vi "Synch with Server.vi"(10 "Sensor File Name":string, 11 "App Config":T1={"Support Dir (Local)"=path "C:/Users/gtetil/Documents/Projects/TI-cDAQ/Source/Support", "Support Dir (Remote)"=path "S:/GLOBALTEST/Software/TI cDAQ/Support", "Config Sub Dir"="Configurations", "Last Config (Std)"="", "Last Config (Def)"="", "Last Config (8TC)"=""}) -> (0 "Error OUT":errorcluster)   [LabVIEW 2023]
uses:
  Type Defs and Controls/App Config.ctl
  Type Defs and Controls/Sensor.ctl
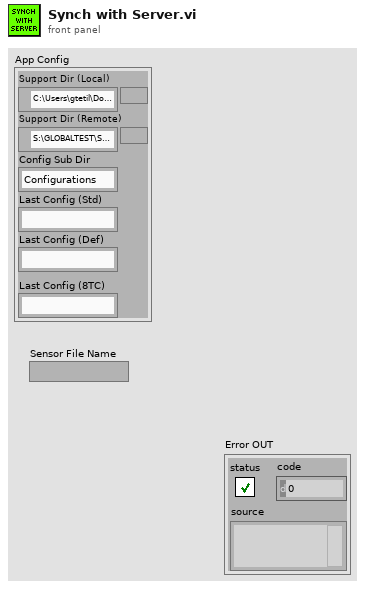
[diagram p1: front panel]
types:
  T1 = typedef "App Config.ctl" = cluster{"Support Dir (Local)":path, "Support Dir (Remote)":path, "Config Sub Dir":string, "Last Config (Std)":string, "Last Config (Def)":string, "Last Config (8TC)":string}
  T2 = typedef "Sensor.ctl" = cluster{"Sensor Name":string, "Sensor Info":cluster{"Manufacturer":string, "Model":string, "Serial Number":string}, "Last Cal Info":cluster{"Last Calibration Date":dbl, "Calibrator":string, "Cal Duration":i32}, "Voltage Range":cluster{"High Limit":dbl, "Low Limit":dbl}, "EGU Range":cluster{"High Limit":dbl, "Low Limit":dbl}, "Units":string, "Calibration Type":enum16{"Calibrate Analog", "Compare Analog Calibration"}, "EGU List":dbl[], "Voltage List":dbl[], "Coefficients":dbl[], "Order":i32, "Algorithm":enum32{"SVD", "Givens", "Givens2", "Householder", "LU Decomposition", "Cholesky"}, "Max Error % of Full Scale":dbl, "Max Mean Squared Error":dbl, "Use Error %":bool, "Use MSE":bool, "Allow Manual Entry":bool, "Max Stability Error":dbl, "Max Error % of Reading":dbl, "Use Error % of Reading":bool}
  T3 = enum16{"Left Button", "Center Button", "Right Button", "Window Close"}
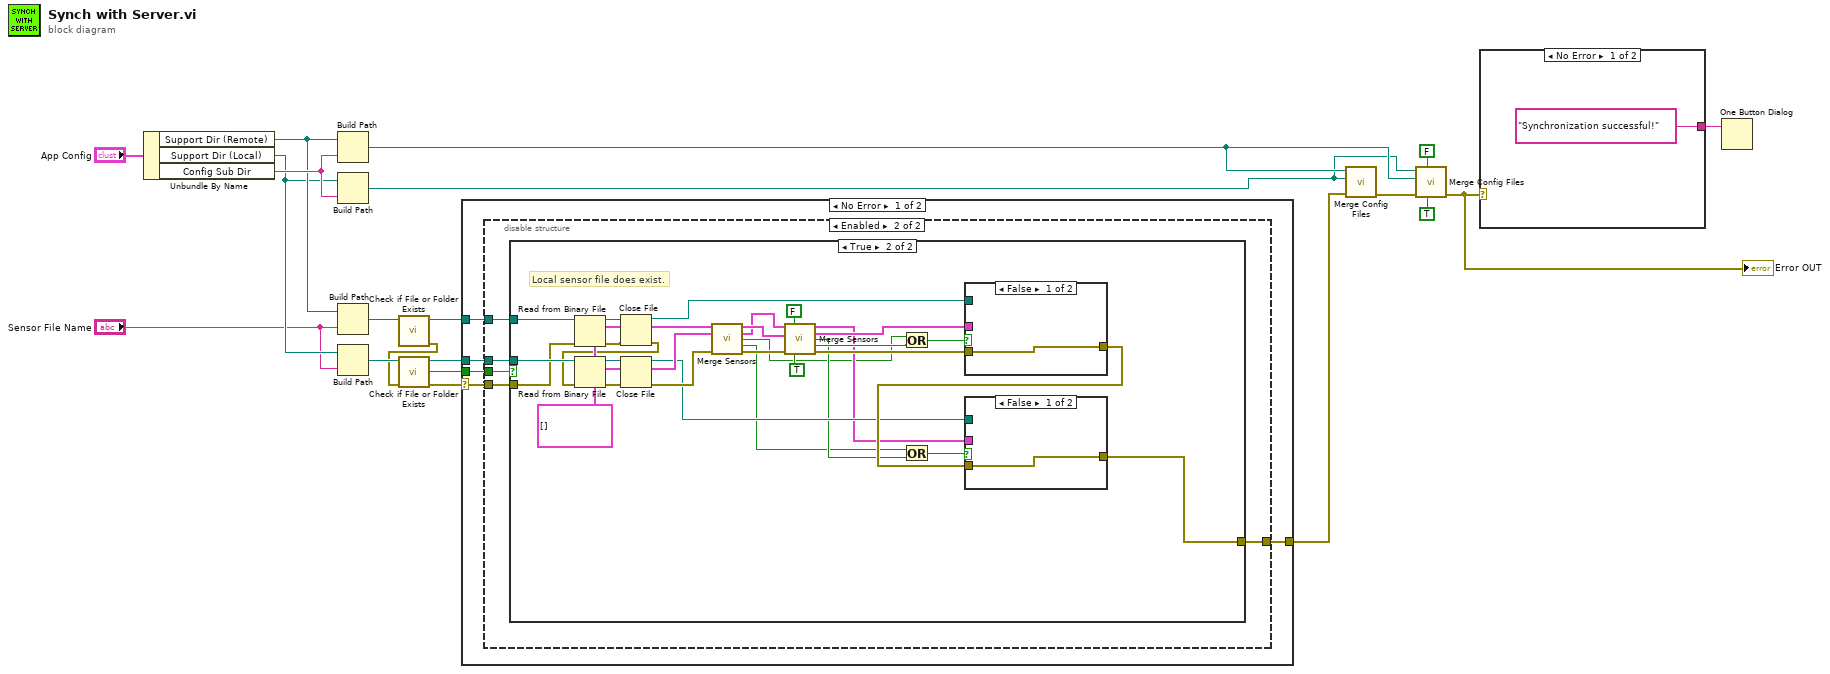
[diagram p0: block diagram]
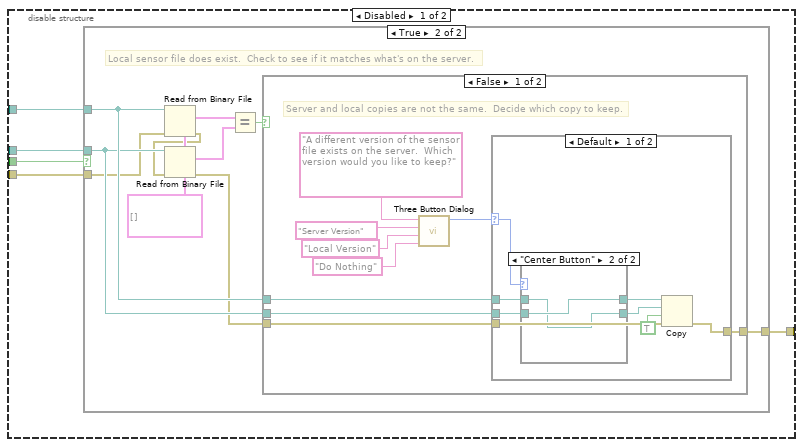
[diagram p2: hidden frame]
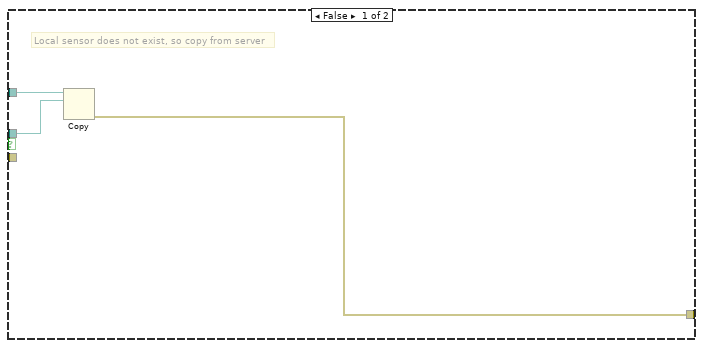
[diagram p3: hidden frame]
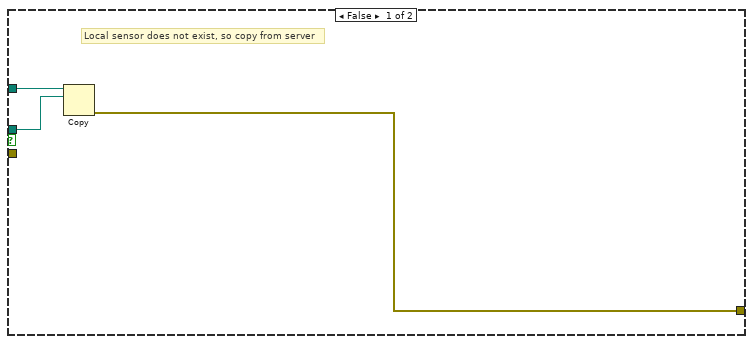
[diagram p7: hidden frame]
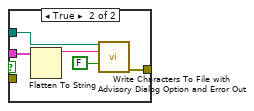
[diagram p8: hidden frame]
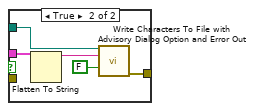
[diagram p9: hidden frame]
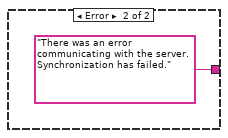
[diagram p11: hidden frame]
diagram:
  n1 = Unbundle By Name("App Config") -> ("Support Dir (Remote)"=w18:path, "Support Dir (Local)"=w17:path, "Config Sub Dir"=w19:string)
  n2 = Build Path(base path=w18, name or relative path=w19) -> (appended path=w15:path)
  n3 = Build Path(base path=w17, name or relative path=w19) -> (appended path=w14:path)
  n4 = Build Path(base path=w18, name or relative path="Sensor File Name") -> (appended path=w4:path)
  n5 = Build Path(base path=w17, name or relative path="Sensor File Name") -> (appended path=w11:path)
  n6 = call <vilib>:"Check if File or Folder Exists.vi"("path"=w4) -> ("error out"=w2:errorcluster, "dup path"=w3:path)  [unwired: 8 in, 1 out]
  n7 = call <vilib>:"Check if File or Folder Exists.vi"("error in (no error)"=w2, "path"=w11) -> ("error out"=w1:errorcluster, "file or folder exists?"=w10:bool, "dup path"=w9:path)  [unwired: 7 in]
  n8 = case shown="No Error" w1 {
    selector: w1 -> [w21 w117]
    tunnel: w10 -> [w25 _]
    tunnel: w9 -> [w24 _]
    tunnel: [w23 w117] -> w6
    tunnel: w3 -> [w22 _]
    frame No Error {
      n9 = disable-structure shown="Enabled" {
        disable-tunnel: w25 -> [w30 w71]
        disable-tunnel: w24 -> [w29 w70]
        disable-tunnel: [w28 w69] -> w23
        disable-tunnel: w22 -> [w27 w68]
        disable-tunnel: w21 -> [w26 w67]
        frame Disabled {
          n10 = case shown="True" w30 {
            tunnel: w27 -> [w33 w39]
            tunnel: w29 -> [w32 w38]
            tunnel: [w31 w37] -> w28
            tunnel: w26 -> [_ w36]
            frame False {
              # "Local sensor does not exist, so copy from server"
              n11 = Copy(10:w32, 11:w33) -> (0:w31:errorcluster)  [unwired: 3 in, 2 out]
            }
            frame True {
              w43 = T2[] [] ("Sensors")
              # "Local sensor file does exist.  Check to see if it matches what's on the server."
              n12 = Read from Binary File(5:w43, 8:w36, 11:w39) -> (0:w35:errorcluster, 2:w42:T2[])  [unwired: 3 in, 2 out]
              n13 = Read from Binary File(5:w43, 8:w35, 11:w38) -> (0:w34:errorcluster, 2:w41:T2[])  [unwired: 3 in, 2 out]
              n14 = Equal?(x=w42, y=w41) -> (x = y?=w40:bool)
              n15 = case shown="False" w40 {
                tunnel: w39 -> [w47 _]
                tunnel: w38 -> [w46 _]
                tunnel: [w45 w66] -> w37
                tunnel: w34 -> [w44 w66]
                frame False {
                  # "Server and local copies are not the same.  Decide which copy to keep."
                  n16 = call <vilib>:"Three Button Dialog.vi"("Right Button Text (\"Cancel\")"="Do Nothing" ("T button name (\"OK\")"), "Center Button Text (\"No\")"="Local Version" ("T button name (\"OK\")"), "Left Button Text (\"Yes\")"="Server Version" ("T button name (\"OK\")"), "message"="A different version of the sensor file exists on the server.  Which version would you like to keep?") -> ("Which Button?"=w48:T3)  [unwired: 7 in]
                  n17 = case shown="Default" w48 {
                    selector: w48 -> [w58 _]
                    tunnel: w47 -> [w57 _]
                    tunnel: [w60 w65] -> w45
                    tunnel: w46 -> [w55 _]
                    tunnel: w44 -> [w53 w65]
                    frame Default {
                      n18 = case shown="\"Center Button\"" w58 {
                        tunnel: [w62 w64] -> w56
                        tunnel: w57 -> [w62 w63]
                        tunnel: [w61 w63] -> w54
                        tunnel: w55 -> [w61 w64]
                        frame "Left Button", Default {
                        }
                        frame "Center Button" {
                        }
                      }
                      n19 = Copy(8:w53, 9:TRUE ("overwrite (F)"), 10:w54, 11:w56) -> (0:w60:errorcluster)  [unwired: 1 in, 2 out]
                    }
                    frame "Right Button" {
                    }
                  }
                }
                frame True {
                  # "Server and local copies are the same, so do nothing."
                }
              }
            }
          }
        }
        frame Enabled {
          n20 = case shown="True" w71 {
            tunnel: w68 -> [w74 w94]
            tunnel: w70 -> [w73 w103]
            tunnel: [w72 w91] -> w69
            tunnel: w67 -> [_ w102]
            frame False {
              # "Local sensor does not exist, so copy from server"
              n21 = Copy(10:w73, 11:w74) -> (0:w72:errorcluster)  [unwired: 3 in, 2 out]
            }
            frame True {
              w104 = T2[] [] ("Sensors")
              # "Local sensor file does exist."
              n22 = Read from Binary File(5:w104, 8:w102, 11:w94) -> (0:w89:errorcluster, 2:w100:T2[], 3:w90:refnum<file>)  [unwired: 3 in, 1 out]
              n23 = Close File(refnum=w90, error in=w89) -> (path=w84:path, error out=w88:errorcluster)
              n24 = Read from Binary File(5:w104, 8:w88, 11:w103) -> (0:w86:errorcluster, 2:w99:T2[], 3:w87:refnum<file>)  [unwired: 3 in, 1 out]
              n25 = Close File(refnum=w87, error in=w86) -> (path=w83:path, error out=w85:errorcluster)
              n26 = call "Merge Sensors.vi"("Source Sensors IN"=w100, "Dest Sensors IN"=w99, "Error IN"=w85) -> ("Source Sensors OUT"=w96:T2[], "Dest Sensors OUT"=w95:T2[], "Source Changed"=w76:bool, "Dest Changed"=w75:bool, "Error OUT"=w101:errorcluster)  [unwired: 8 in]
              n27 = call "Merge Sensors.vi"("Source Sensors IN"=w95, "Server is Source (T)"=FALSE, "Dest Sensors IN"=w96, "Error IN"=w101, "Version Prompt (F)"=TRUE) -> ("Source Sensors OUT"=w77:T2[], "Dest Sensors OUT"=w78:T2[], "Source Changed"=w79:bool, "Dest Changed"=w80:bool, "Error OUT"=w93:errorcluster)  [unwired: 6 in]
              n28 = Or(x=w76, y=w80) -> (x .or. y?=w82:bool)
              n29 = Or(x=w75, y=w79) -> (x .or. y?=w81:bool)
              n30 = case shown="False" w82 {
                tunnel: w78 -> [_ w113]
                tunnel: w93 -> [w111 _]
                tunnel: [w111 w112] -> w92
                tunnel: w84 -> [_ w114]
                frame False {
                }
                frame True {
                  n31 = Flatten To String(anything=w113) -> (data string=w116:string)  [unwired: 3 in, 2 out]
                  n32 = call "Write Characters To File with Advisory Dialog Option and Error Out.vi"("file path (dialog if empty)"=w114, "character string"=w116, "advisory dialog? (display:T)"=FALSE) -> ("error out"=w112:errorcluster)  [unwired: 11 in, 1 out]
                }
              }
              n33 = case shown="False" w81 {
                tunnel: w92 -> [w105 _]
                tunnel: [w105 w108] -> w91
                tunnel: w77 -> [_ w106]
                tunnel: w83 -> [_ w107]
                frame False {
                }
                frame True {
                  n34 = Flatten To String(anything=w106) -> (data string=w109:string)  [unwired: 3 in, 2 out]
                  n35 = call "Write Characters To File with Advisory Dialog Option and Error Out.vi"("file path (dialog if empty)"=w107, "character string"=w109, "advisory dialog? (display:T)"=FALSE) -> ("error out"=w108:errorcluster)  [unwired: 11 in, 1 out]
                }
              }
            }
          }
        }
      }
    }
    frame Error {
    }
  }
  n36 = call "Merge Config Files.vi"("Error IN"=w6, "Dest Path"=w14, "Source Path"=w15) -> ("Error OUT"=w12:errorcluster)  [unwired: 8 in]
  n37 = call "Merge Config Files.vi"("Version Prompt (F)"=TRUE, "Server is Source (T)"=FALSE, "Error IN"=w12, "Dest Path"=w15, "Source Path"=w14) -> ("Error OUT"=w5:errorcluster)  [unwired: 6 in]
  "Error OUT" <- w5
  n38 = case shown="No Error" w5 {
    tunnel: ["Synchronization successful!" ("message") "There was an error communicating with the server.  Synchronization has failed." ("message")] -> w8
    frame No Error {
    }
    frame Error {
    }
  }
  n39 = One Button Dialog(message=w8) -> ()  [unwired: 1 in, 1 out]
